vi "SizeDown.vi"() -> ()   [LabVIEW 2024, in "TypedCircularBuffer.Tests.Units.lvlib"]
uses:
  TypedCircularBuffer.Tests.Units.lvlib
  <vilib>/addons/_JKI Toolkits/Caraya/classes/Test/Test.lvclass
  TypedCircularBuffer.lvclass
  <vilib>/addons/_JKI Toolkits/Caraya/classes/Assert/Assert.lvclass
  <vilib>/addons/_JKI Toolkits/Caraya/classes/Assert/Assert True.vi
  <vilib>/addons/_JKI Toolkits/Caraya/classes/Assert/Assert Equal Value_Variant.vi
  Type.ctl
panel:
  in  "Size down Add Expected 7":T1[](array[typedef])=[5, 6, 7, 8, 9, 10, 255]
  in  "Size down Expected 7":T1[](array[typedef])=[4, 5, 6, 7, 8, 9, 10]
  in  "Size down Add Expected 3":T1[](array[typedef])=[9, 10, 255]
  in  "Size down Expected 3":T1[](array[typedef])=[8, 9, 10]
  in  "Size down Add Expected":T1[](array[typedef])=[7, 8, 9, 10, 255]
  in  "Size down Expected":T1[](array[typedef])=[6, 7, 8, 9, 10]
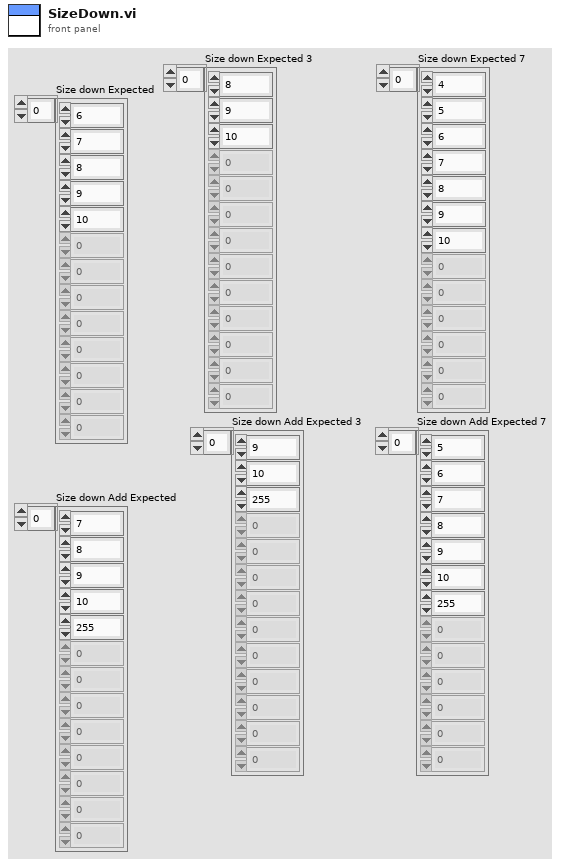
[diagram p1: front panel]
types:
  T1 = typedef "TypedCircularBuffer.lvclass/Type.ctl" = i32
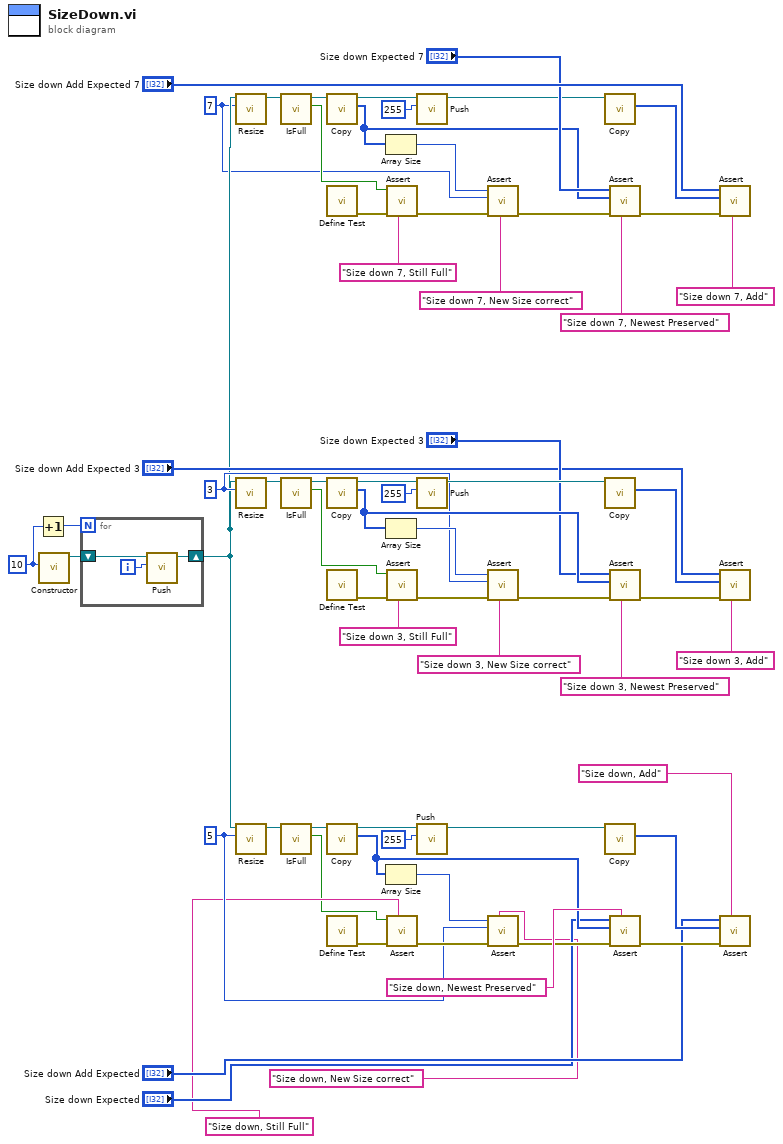
[diagram p0: block diagram]
diagram:
  w5 = u32 7 ("Capacity")
  w24 = u32 3 ("Capacity")
  w51 = u32 5 ("Capacity")
  w44 = u32 10 ("Capacity")
  n1 = Increment(x=w44) -> (x+1=w43:u32)
  n2 = call "Constructor.vi"("Capacity"=w44) -> ("TypedCircularBuffer out"=w42:refnum<class "TypedCircularBuffer.lvclass">)  [unwired: 10 in]
  n3 = for {
    N: w43 -> [_]
    shift-right: [w66] -> w6
    shift-left: w42 -> [w67]
    i -> [w65]
    n4 = call "Push.vi"("Element"=w65, "TypedCircularBuffer in"=w67) -> ("TypedCircularBuffer out"=w66:refnum<class "TypedCircularBuffer.lvclass">)  [unwired: 7 in, 2 out]
  }
  n5 = call "Resize.vi"("Capacity"=w5, "TypedCircularBuffer in"=w6) -> ("TypedCircularBuffer out"=w7:refnum<class "TypedCircularBuffer.lvclass">)  [unwired: 9 in]
  n6 = call "Resize.vi"("Capacity"=w24, "TypedCircularBuffer in"=w6) -> ("TypedCircularBuffer out"=w41:refnum<class "TypedCircularBuffer.lvclass">)  [unwired: 9 in]
  n7 = call "Resize.vi"("Capacity"=w51, "TypedCircularBuffer in"=w6) -> ("TypedCircularBuffer out"=w45:refnum<class "TypedCircularBuffer.lvclass">)  [unwired: 9 in]
  n8 = call "IsFull.vi"("TypedCircularBuffer in"=w7) -> ("Full?"=w9:bool, "TypedCircularBuffer out"=w10:refnum<class "TypedCircularBuffer.lvclass">)  [unwired: 9 in]
  n9 = call "IsFull.vi"("TypedCircularBuffer in"=w41) -> ("Full?"=w39:bool, "TypedCircularBuffer out"=w37:refnum<class "TypedCircularBuffer.lvclass">)  [unwired: 9 in]
  n10 = call "IsFull.vi"("TypedCircularBuffer in"=w45) -> ("Full?"=w47:bool, "TypedCircularBuffer out"=w49:refnum<class "TypedCircularBuffer.lvclass">)  [unwired: 9 in]
  n11 = call "Copy.vi"("TypedCircularBuffer in"=w10) -> ("Copied Buffer"=w13:T1[], "TypedCircularBuffer out"=w15:refnum<class "TypedCircularBuffer.lvclass">)  [unwired: 9 in]
  n12 = call <vilib>:"Define Test.vi"() -> ("error out"=w8:errorcluster)  [unwired: 10 in, 1 out]
  n13 = call "Copy.vi"("TypedCircularBuffer in"=w37) -> ("Copied Buffer"=w33:T1[], "TypedCircularBuffer out"=w30:refnum<class "TypedCircularBuffer.lvclass">)  [unwired: 9 in]
  n14 = call <vilib>:"Define Test.vi"() -> ("error out"=w40:errorcluster)  [unwired: 10 in, 1 out]
  n15 = call "Copy.vi"("TypedCircularBuffer in"=w49) -> ("Copied Buffer"=w55:T1[], "TypedCircularBuffer out"=w58:refnum<class "TypedCircularBuffer.lvclass">)  [unwired: 9 in]
  n16 = call <vilib>:"Define Test.vi"() -> ("error out"=w46:errorcluster)  [unwired: 10 in, 1 out]
  n17 = Array Size(array=w13) -> (size(s)=w11:i32)
  n18 = Array Size(array=w33) -> (size(s)=w36:i32)
  n19 = Array Size(array=w55) -> (size(s)=w50:i32)
  n20 = call-poly <vilib>:"Assert.vi"("Label"="Size down 7, Still Full", "error in (no error)"=w8, "True?"=w9) -> ("error out"=w12:errorcluster)  [unwired: 7 in, 1 out]
  n21 = call-poly <vilib>:"Assert.vi"("Label"="Size down 3, Still Full", "error in (no error)"=w40, "True?"=w39) -> ("error out"=w34:errorcluster)  [unwired: 7 in, 1 out]
  n22 = call-poly <vilib>:"Assert.vi"("Label"="Size down, Still Full", "error in (no error)"=w46, "True?"=w47) -> ("error out"=w53:errorcluster)  [unwired: 7 in, 1 out]
  n23 = call "Push.vi"("Element"=u8 255, "TypedCircularBuffer in"=w15) -> ("TypedCircularBuffer out"=w19:refnum<class "TypedCircularBuffer.lvclass">)  [unwired: 7 in, 2 out]
  n24 = call "Push.vi"("Element"=u8 255, "TypedCircularBuffer in"=w30) -> ("TypedCircularBuffer out"=w25:refnum<class "TypedCircularBuffer.lvclass">)  [unwired: 7 in, 2 out]
  n25 = call "Push.vi"("Element"=u8 255, "TypedCircularBuffer in"=w58) -> ("TypedCircularBuffer out"=w60:refnum<class "TypedCircularBuffer.lvclass">)  [unwired: 7 in, 2 out]
  n26 = call-poly <vilib>:"Assert.vi"("Label"="Size down 7, New Size correct", "error in (no error)"=w12, "Y"=w5, "X"=w11) -> ("error out"=w14:errorcluster)  [unwired: 6 in, 1 out]
  n27 = call-poly <vilib>:"Assert.vi"("Label"="Size down 3, New Size correct", "error in (no error)"=w34, "Y"=w24, "X"=w36) -> ("error out"=w32:errorcluster)  [unwired: 6 in, 1 out]
  n28 = call-poly <vilib>:"Assert.vi"("Label"="Size down, New Size correct", "error in (no error)"=w53, "Y"=w51, "X"=w50) -> ("error out"=w56:errorcluster)  [unwired: 6 in, 1 out]
  n29 = call "Copy.vi"("TypedCircularBuffer in"=w19) -> ("Copied Buffer"=w17:T1[])  [unwired: 9 in, 1 out]
  n30 = call "Copy.vi"("TypedCircularBuffer in"=w25) -> ("Copied Buffer"=w28:T1[])  [unwired: 9 in, 1 out]
  n31 = call "Copy.vi"("TypedCircularBuffer in"=w60) -> ("Copied Buffer"=w62:T1[])  [unwired: 9 in, 1 out]
  n32 = call-poly <vilib>:"Assert.vi"("Label"="Size down 7, Newest Preserved", "error in (no error)"=w14, "Y"=w13, "X"="Size down Expected 7") -> ("error out"=w18:errorcluster)  [unwired: 6 in, 1 out]
  n33 = call-poly <vilib>:"Assert.vi"("Label"="Size down 3, Newest Preserved", "error in (no error)"=w32, "Y"=w33, "X"="Size down Expected 3") -> ("error out"=w26:errorcluster)  [unwired: 6 in, 1 out]
  n34 = call-poly <vilib>:"Assert.vi"("Label"="Size down, Newest Preserved", "error in (no error)"=w56, "Y"=w55, "X"="Size down Expected") -> ("error out"=w64:errorcluster)  [unwired: 6 in, 1 out]
  n35 = call-poly <vilib>:"Assert.vi"("Label"="Size down 7, Add", "error in (no error)"=w18, "Y"=w17, "X"="Size down Add Expected 7") -> ()  [unwired: 6 in, 2 out]
  n36 = call-poly <vilib>:"Assert.vi"("Label"="Size down 3, Add", "error in (no error)"=w26, "Y"=w28, "X"="Size down Add Expected 3") -> ()  [unwired: 6 in, 2 out]
  n37 = call-poly <vilib>:"Assert.vi"("Label"="Size down, Add", "error in (no error)"=w64, "Y"=w62, "X"="Size down Add Expected") -> ()  [unwired: 6 in, 2 out]
